vi "Frequency Response (Mag-Phase).vi"(0 "scaled signal X [EUx]":dbl[](array[numeric]) format="%.2f", 1 "scaled signal Y [EUy]":dbl[](array[numeric]) format="%.2f", 2 "sampling frequency [Hz]":dbl=10000.0 format="%.2f", 3 "view":T5, 4 "channel X info":T2={"sensor sensitivity [mV/EU]"=1000.0, "engineering units"=1, "dB reference [EU]"=1.0, "custom label"="EU", "weighting filter"=0, "pregain [dB]"=0.0} {"pregain [dB]" format="%.2f"; "weighting filter" items=["Linear", "A-weighting", "B-weighting", "C-weighting", "ITU-R 468-4", "Dolby", "CCITT", "C-message"]; "dB reference [EU]" format="%^.1e"; "engineering units" items=["custom..."=0, "V"=1, "A"=21, "Pa"=2, "N"=20, "g"=3, "m/s^2"=4, "m/s"=5, "m"=6, "mm/s"=12, "mm"=13, "microns/s"=14, "microns"=15, "in/s^2"=7, "in/s"=8, "in"=9, "mils/s"=10, "mils"=11, "rad/s^2"=16, "rad/s"=17, "rad"=18, "strain"=19]; "sensor sensitivity [mV/EU]" format="%.2f"}, 5 "channel Y info":T2={"sensor sensitivity [mV/EU]"=1000.0, "engineering units"=1, "dB reference [EU]"=1.0, "custom label"="EU", "weighting filter"=0, "pregain [dB]"=0.0} {"pregain [dB]" format="%.2f"; "weighting filter" items=["Linear", "A-weighting", "B-weighting", "C-weighting", "ITU-R 468-4", "Dolby", "CCITT", "C-message"]; "dB reference [EU]" format="%^.1e"; "engineering units" items=["custom..."=0, "V"=1, "A"=21, "Pa"=2, "N"=20, "g"=3, "m/s^2"=4, "m/s"=5, "m"=6, "mm/s"=12, "mm"=13, "microns/s"=14, "microns"=15, "in/s^2"=7, "in/s"=8, "in"=9, "mils/s"=10, "mils"=11, "rad/s^2"=16, "rad/s"=17, "rad"=18, "strain"=19]; "sensor sensitivity [mV/EU]" format="%.2f"}, 6 "window":T7=1 items=["None"=0, "Hanning"=1, "Hamming"=2, "Blackman-Harris"=3, "Exact Blackman"=4, "Blackman"=5, "Flat Top"=6, "4 Term B-Harris "=7, "7 Term B-Harris"=8, "Low Sidelobe"=9, "Force - Exponential"=10, "Blackman Nuttall"=11, "Triangle"=30, "Bartlett-Hanning"=31, "Bohman"=32, "Parzen"=33, "Welch"=34, "Kaiser"=60, "Dolph-Chebyshev"=61, "Gaussian"=62], 7 "reset averaging (T)":bool=TRUE, 8 "force/exp settings":T6={"force window [%]"=50.0, "exponential window [%]"=10.0} {"exponential window [%]" min=0.0 max=100.0 format="%.2f"; "force window [%]" min=0.0 max=100.0 format="%.2f"}, 9 "averaging parameters":T1={"averaging mode"=enum."RMS averaging", "weighting mode"=enum."Linear", "number of averages"=10} {"number of averages" min=1}, 10 "FRF mode":enum16{"H1", "H2", "H3"}(ring)) -> (11 "window constants":cluster{"eq noise BW":dbl, "coherent gain":dbl} {"coherent gain" format="%.2f"; "eq noise BW" format="%.2f"}, 12 "df [Hz]":dbl format="%.2f", 13 "averages completed":dbl format="%.2f", 14 "magnitude [EUy/EUx rms]":dbl[](array[numeric]) format="%.2f", 15 "unit label (magnitude)":string, 16 "phase":dbl[](array[numeric]) format="%.2f", 17 "unit label (phase)":string, 18 "coherence":dbl[](array[numeric]) format="%.2f", 19 "error out":errorcluster)   [LabVIEW 2017]
doc: "Computes the frequency response and the coherence based on the input signals. Typically, X signal is the stimulus, and Y signal is the response of the system. Results are returned as magnitude and phase.\nFrequency response is typically an averaged measurement. Each block of data corresponds to a single FFT block and must be passed individually to this VI. The first time this VI is called, reset averaging must be TRUE (default value), to start a new averaging process. For subsequent calls, reset averaging must be FALSE to continue the averaging process. Averages completed returns the number of averages completed so far.\nAveraging parameters specifies how the averaging is performed. This includes the averaging mode (no averaging, vector averaging, or RMS averaging), the weighting mode (linear or exponential), and the number of averages (used only if the weighting mode is exponential).\nThe view cluster allows you to display magnitude results in decibels or not, and the phase results unwrapped or not, in radians or degrees."
uses:
  <vilib>/addons/_NISVFA/_Shared subVIs/Controls/svc_Window [Dual FFT].ctl
  <vilib>/addons/Sound and Vibration/compatibility/Controls/svl_Channel Info.ctl
  <vilib>/addons/Sound and Vibration/compatibility/Controls/svl_Engineering Units Text Ring.ctl
  <vilib>/addons/Sound and Vibration/compatibility/Controls/svl_Weighting Filter Text Ring.ctl
  <vilib>/Analysis/4window.llb/Force Window (DBL).vi
  <vilib>/Analysis/4window.llb/Exponential Window (DBL).vi
  <vilib>/Analysis/2dsp.llb/Real FFT.vi
  <vilib>/Analysis/2dsp.llb/Power Spectrum (DBL).vi
  <vilib>/Analysis/2dsp.llb/Cross Power (DBL).vi
  <vilib>/Analysis/0measdsp.llb/Scaled Time Domain Window (DBL).vi
  <vilib>/Analysis/NI_AALPro.lvlib
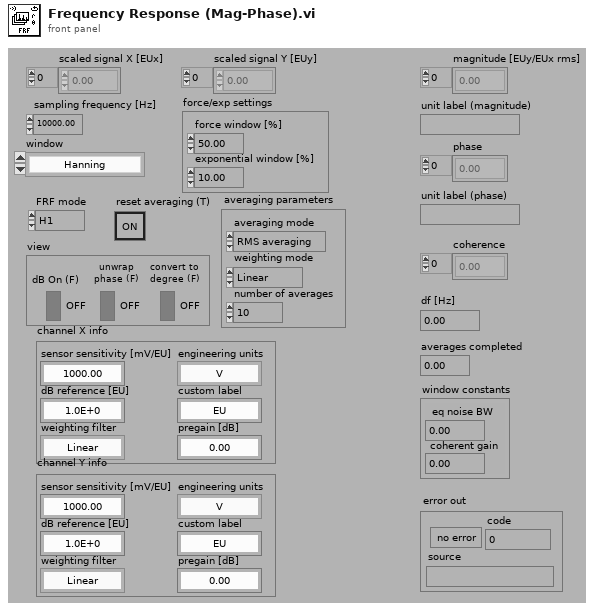
[diagram p1: front panel]
types:
  T1 = cluster{"averaging mode":enum16{"No averaging", "Vector averaging", "RMS averaging"}, "weighting mode":enum16{"Linear", "Exponential"}, "number of averages":u32}
  T2 = typedef "svl_Channel Info.ctl" = cluster{"sensor sensitivity [mV/EU]":dbl, "engineering units":T3, "dB reference [EU]":dbl, "custom label":string, "weighting filter":T4, "pregain [dB]":dbl}
  T3 = typedef "svl_Engineering Units Text Ring.ctl" = u16
  T4 = typedef "svl_Weighting Filter Text Ring.ctl" = u16
  T5 = cluster{"dB On (F)":bool, "unwrap phase (F)":bool, "convert to degree (F)":bool}
  T6 = cluster{"force window [%]":dbl, "exponential window [%]":dbl}
  T7 = typedef "svc_Window [Dual FFT].ctl" = u32
  T8 = enum16{"No averaging", "Vector averaging", "RMS averaging"}
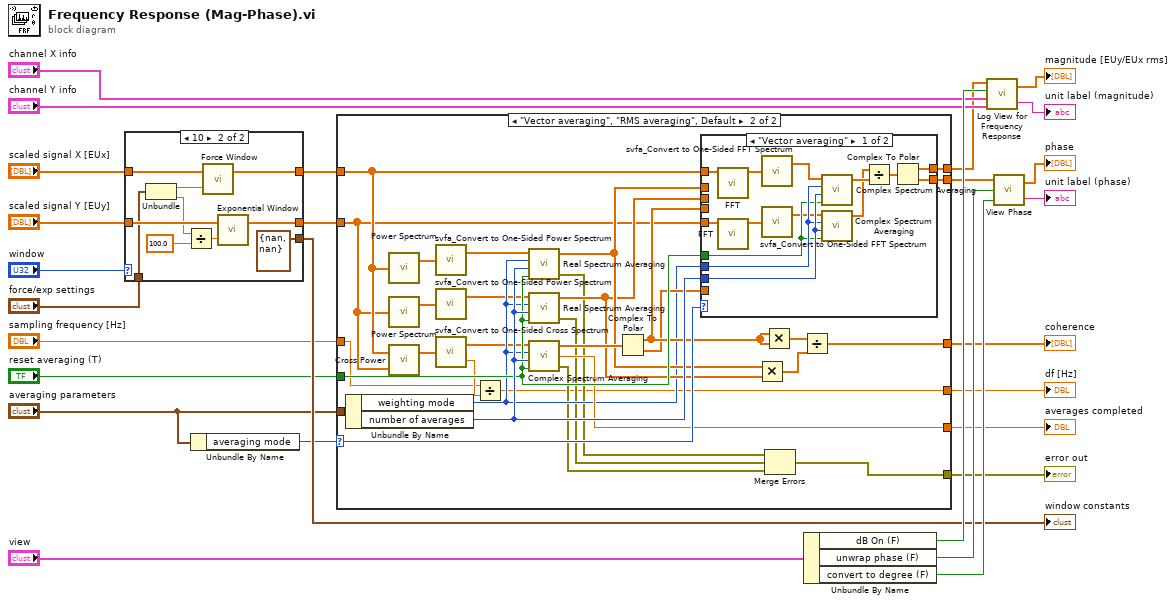
[diagram p0: block diagram]
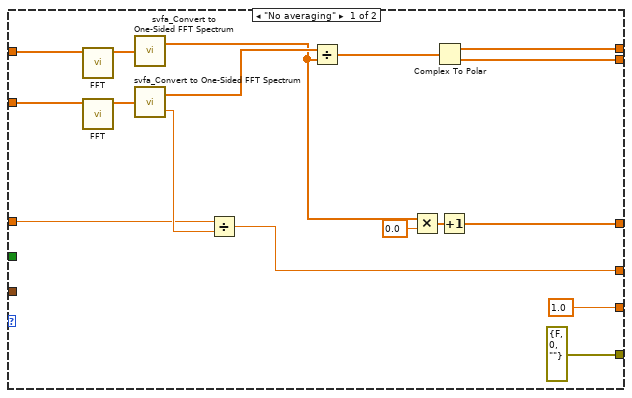
[diagram p2: hidden frame]
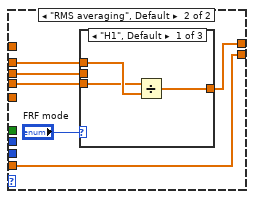
[diagram p3: hidden frame]
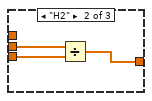
[diagram p4: hidden frame]
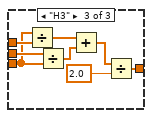
[diagram p5: hidden frame]
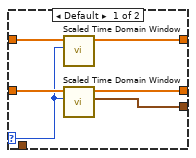
[diagram p6: hidden frame]
diagram:
  n1 = case shown="10" "window" {
    selector: "window" -> [w28 _]
    tunnel: "scaled signal X [EUx]" -> [w33 w43]
    tunnel: "scaled signal Y [EUy]" -> [w32 w42]
    tunnel: "force/exp settings" -> [_ w38]
    tunnel: [w31 w40] -> w14
    tunnel: [w30 w39] -> w13
    tunnel: [w29 cluster{"eq noise BW":dbl, "coherent gain":dbl} {"eq noise BW"=nan, "coherent gain"=nan} ("window constants")] -> w15
    frame Default {
      n2 = call-poly <vilib>:"Scaled Time Domain Window.vi"("window"=w28, "X"=w33) -> ("Windowed X"=w31:dbl[])  [unwired: 7 in, 2 out]
      n3 = call-poly <vilib>:"Scaled Time Domain Window.vi"("window"=w28, "X"=w32) -> ("window properties"=w29:cluster{"eq noise BW":dbl, "coherent gain":dbl}, "Windowed X"=w30:dbl[])  [unwired: 7 in, 1 out]
    }
    frame 10 {
      n4 = Unbundle(w38) -> ("force window [%]"=w37:dbl, "exponential window [%]"=w36:dbl)
      n5 = Divide(x=w36, y=100.0 ("x")) -> (x/y=w41:dbl)
      n6 = call-poly <vilib>:"Force Window.vi"("duty cycle(%)"=w37, "X"=w43) -> ("Windowed X"=w40:dbl[])  [unwired: 1 out]
      n7 = call-poly <vilib>:"Exponential Window.vi"("final value"=w41, "X"=w42) -> ("Windowed X"=w39:dbl[])  [unwired: 1 out]
    }
  }
  "window constants" <- w15
  n8 = Unbundle By Name("averaging parameters") -> ("averaging mode"=w9:T8)
  n9 = case shown="\"Vector averaging\", \"RMS averaging\", Default" w9 {
    selector: w9 -> [_ w87]
    tunnel: w14 -> [w53 w65]
    tunnel: "sampling frequency [Hz]" -> [w49 w68]
    tunnel: [w48 w61] -> w8
    tunnel: "reset averaging (T)" -> [_ w85]
    tunnel: "averaging parameters" -> [_ w91]
    tunnel: [1.0 ("averages completed") w77] -> w7
    tunnel: w13 -> [w52 w63]
    tunnel: [w44 w84] -> w6
    tunnel: [w58 w83] -> w5
    tunnel: [w57 w82] -> w4
    tunnel: [errorcluster {"status"=FALSE, "code"=0, "source"=""} ("error out") w72] -> w1
    frame "No averaging" {
      n10 = call-poly <vilib>:"FFT.vi"("X"=w53) -> ("FFT {X}"=w55:cdb[])  [unwired: 9 in, 1 out]
      n11 = call-poly <vilib>:"FFT.vi"("X"=w52) -> ("FFT {X}"=w54:cdb[])  [unwired: 9 in, 1 out]
      n12 = call <vilib>:"svfa_Convert to One-Sided FFT Spectrum.vi"("two-sided FFT spectrum"=w55) -> ("one-sided FFT spectrum"=w47:cdb[])  [unwired: 1 out]
      n13 = call <vilib>:"svfa_Convert to One-Sided FFT Spectrum.vi"("two-sided FFT spectrum"=w54) -> ("one-sided FFT spectrum"=w51:cdb[], "block size"=w50:dbl)
      n14 = Divide(x=w49, y=w50) -> (x/y=w48:dbl)
      n15 = Divide(x=w51, y=w47) -> (x/y=w59:cdb[])
      n16 = Multiply(x=w47, y=0.0) -> (x*y=w45:cdb[])
      n17 = Complex To Polar(r * e^(i*theta)=w59) -> (r=w58:dbl[], theta=w57:dbl[])
      n18 = Increment(x=w45) -> (x+1=w44:cdb[])
    }
    frame "Vector averaging", "RMS averaging", Default {
      n19 = Unbundle By Name(w91) -> ("weighting mode"=w76:enum16{"Linear", "Exponential"}, "number of averages"=w86:u32)
      n20 = call-poly <vilib>:"Power Spectrum.vi"("X"=w65) -> ("Power Spectrum"=w67:dbl[])  [unwired: 1 out]
      n21 = call-poly <vilib>:"Power Spectrum.vi"("X"=w63) -> ("Power Spectrum"=w66:dbl[])  [unwired: 1 out]
      n22 = call-poly <vilib>:"Cross Power.vi"("Y"=w63, "X"=w65) -> ("Sxy"=w71:cdb[])  [unwired: 1 out]
      n23 = call <vilib>:"svfa_Convert to One-Sided Power Spectrum.vi"("two-sided power spectrum"=w67) -> ("one-sided power spectrum"=w64:dbl[])  [unwired: 1 out]
      n24 = call <vilib>:"svfa_Convert to One-Sided Power Spectrum.vi"("two-sided power spectrum"=w66) -> ("one-sided power spectrum"=w62:dbl[])  [unwired: 1 out]
      n25 = call <vilib>:"svfa_Convert to One-Sided Cross Spectrum.vi"("two-sided cross spectrum"=w71) -> ("one-sided cross spectrum"=w70:cdb[], "block size"=w69:dbl)
      n26 = Divide(x=w68, y=w69) -> (x/y=w61:dbl)
      n27 = call <vilib>:"Real Spectrum Averaging.vi"("reset averaging (T)"=w85, "number of averages"=w86, "weighting mode"=w76, "real spectrum"=w64) -> ("error out"=w75:errorcluster, "averaged real spectrum"=w80:dbl[])  [unwired: 1 out]
      n28 = call <vilib>:"Real Spectrum Averaging.vi"("reset averaging (T)"=w85, "number of averages"=w86, "weighting mode"=w76, "real spectrum"=w62) -> ("error out"=w74:errorcluster, "averaged real spectrum"=w79:dbl[])  [unwired: 1 out]
      n29 = call <vilib>:"Complex Spectrum Averaging.vi"("reset averaging (T)"=w85, "number of averages"=w86, "weighting mode"=w76, "complex spectrum"=w70) -> ("error out"=w73:errorcluster, "averages completed"=w77:dbl, "averaged complex spectrum"=w90:cdb[])
      n30 = Complex To Polar(r * e^(i*theta)=w90) -> (r=w81:dbl[], theta=w78:dbl[])
      n31 = case shown="\"Vector averaging\"" w87 {
        tunnel: w65 -> [w93 _]
        tunnel: w63 -> [w96 _]
        tunnel: w86 -> [w103 _]
        tunnel: w76 -> [w102 _]
        tunnel: w85 -> [w101 _]
        tunnel: [w99 w107] -> w83
        tunnel: [w98 w106] -> w82
        tunnel: w81 -> [_ w110]
        tunnel: w80 -> [_ w109]
        tunnel: w79 -> [_ w108]
        tunnel: w78 -> [_ w106]
        frame "Vector averaging" {
          n32 = call-poly <vilib>:"FFT.vi"("X"=w93) -> ("FFT {X}"=w94:cdb[])  [unwired: 9 in, 1 out]
          n33 = call-poly <vilib>:"FFT.vi"("X"=w96) -> ("FFT {X}"=w97:cdb[])  [unwired: 9 in, 1 out]
          n34 = call <vilib>:"svfa_Convert to One-Sided FFT Spectrum.vi"("two-sided FFT spectrum"=w94) -> ("one-sided FFT spectrum"=w92:cdb[])  [unwired: 1 out]
          n35 = call <vilib>:"svfa_Convert to One-Sided FFT Spectrum.vi"("two-sided FFT spectrum"=w97) -> ("one-sided FFT spectrum"=w95:cdb[])  [unwired: 1 out]
          n36 = call <vilib>:"Complex Spectrum Averaging.vi"("reset averaging (T)"=w101, "number of averages"=w103, "weighting mode"=w102, "complex spectrum"=w92) -> ("averaged complex spectrum"=w105:cdb[])  [unwired: 2 out]
          n37 = call <vilib>:"Complex Spectrum Averaging.vi"("reset averaging (T)"=w101, "number of averages"=w103, "weighting mode"=w102, "complex spectrum"=w95) -> ("averaged complex spectrum"=w104:cdb[])  [unwired: 2 out]
          n38 = Divide(x=w104, y=w105) -> (x/y=w100:cdb[])
          n39 = Complex To Polar(r * e^(i*theta)=w100) -> (r=w99:dbl[], theta=w98:dbl[])
        }
        frame "RMS averaging", Default {
          n40 = case shown="\"H1\", Default" "FRF mode" {
            tunnel: w109 -> [w114 _ w124]
            tunnel: [w113 w116 w125] -> w107
            tunnel: w108 -> [_ w117 w123]
            tunnel: w110 -> [w112 w115 w118]
            frame "H1", Default {
              n41 = Divide(x=w112, y=w114) -> (x/y=w113:dbl[])
            }
            frame "H2" {
              n42 = Divide(x=w117, y=w115) -> (x/y=w116:dbl[])
            }
            frame "H3" {
              n43 = Divide(x=w118, y=w124) -> (x/y=w119:dbl[])
              n44 = Divide(x=w123, y=w118) -> (x/y=w120:dbl[])
              n45 = Add(x=w119, y=w120) -> (x+y=w121:dbl[])
              n46 = Divide(x=w121, y=2.0) -> (x/y=w125:dbl[])
            }
          }
        }
      }
      n47 = Multiply(x=w80, y=w79) -> (x*y=w88:dbl[])
      n48 = Multiply(x=w81, y=w81) -> (x*y=w89:dbl[])
      n49 = Merge Errors(w75, w74, w73) -> (w72:errorcluster)
      n50 = Divide(x=w89, y=w88) -> (x/y=w84:dbl[])
    }
  }
  "df [Hz]" <- w8
  "averages completed" <- w7
  "coherence" <- w6
  "error out" <- w1
  n51 = Unbundle By Name("view") -> ("dB On (F)"=w18:bool, "unwrap phase (F)"=w20:bool, "convert to degree (F)"=w19:bool)
  n52 = call <vilib>:"Log View for Frequency Response.vi"("channel Y info"="channel Y info", "channel X info"="channel X info", "dB On (T)"=w18, "FRF [EUy/EUx]"=w5) -> ("unit label"=→"unit label (magnitude)":string, "log view FRF [dB EUy/EUx]"=→"magnitude [EUy/EUx rms]":dbl[])
  n53 = call <vilib>:"View Phase.vi"("convert to degree (F)"=w19, "unwrap phase (F)"=w20, "phase (radian)"=w4) -> ("unit label (phase)"=→"unit label (phase)":string, "scaled phase"=→"phase":dbl[])
